vi "xml_set_target.vi"(2 "error in (no error)":errorcluster, 3 "XML Path":path=path "D:/Test Management/Farmer/XML/targets.xml", 4 "Data":T1) -> (0 "error out":errorcluster, 1 "success?":bool)   [LabVIEW 2011]
uses:
  TargetData.ctl
  <vilib>/xml/Load XML File.vi
  <vilib>/xml/Close Reference(Node).vi
  <vilib>/xml/NI_XML.lvlib
  Program Files/National Instruments/LabVIEW 2011/resource/objmgr/DOMUserDefRef.rc
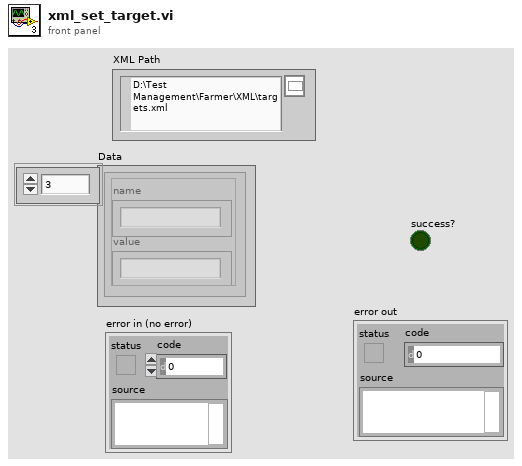
[diagram p1: front panel]
types:
  T1 = typedef "TargetData.ctl" = cluster{"name":string, "value":string}[]
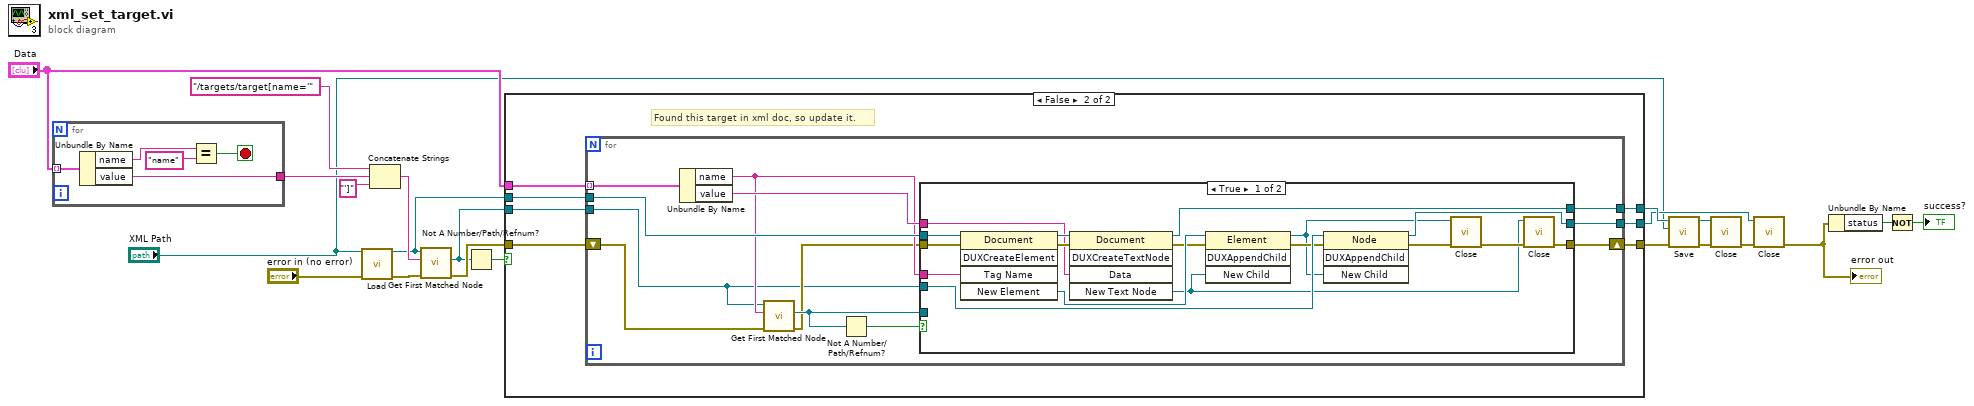
[diagram p0: block diagram]
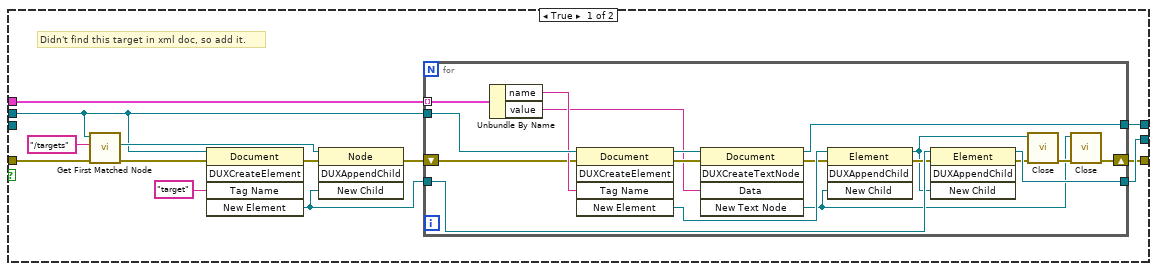
[diagram p2: hidden frame]
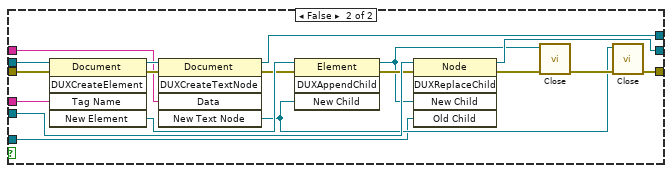
[diagram p3: hidden frame]
diagram:
  n1 = for {
    tunnel: "Data" -> [w26] mode=indexing
    tunnel: [w22] -> w14
    stop <- w23 stop-if-true
    n2 = Unbundle By Name(w26) -> ("name"=w25:string, "value"=w22:string)
    n3 = Equal?(x=w25, y="name") -> (x = y?=w23:bool)
  }
  n4 = call-poly <vilib>:"Load.vi"("path to XML document"="XML Path", "error in (no error)"="error in (no error)") -> ("DOM document out"=w15:refnum<k20>, "error out"=w18:errorcluster)  [unwired: 11 in, 1 out]
  n5 = Concatenate Strings("/targets/target[name='", w14, "']") -> (w19:string)
  n6 = call <vilib>:"Get First Matched Node.vi"("error in (no error)"=w18, "XPath expression"=w19, "node in"=w15) -> ("error out"=w17:errorcluster, "node result"=w6:refnum<k20>)  [unwired: 6 in, 1 out]
  n7 = Not A Number/Path/Refnum?(number/path/refnum=w6) -> (NaN/Path/Refnum?=w16:bool)
  n8 = case shown="False" w16 {
    tunnel: w17 -> [w36 w60]
    tunnel: w15 -> [w29 w63]
    tunnel: "Data" -> [w38 w64]
    tunnel: [w27 w61] -> w12
    tunnel: [w28 w62] -> w11
    tunnel: [w30 w58] -> w10
    tunnel: w6 -> [_ w59]
    frame True {
      # "Didn't find this target in xml doc, so add it."
      n9 = call <vilib>:"Get First Matched Node.vi"("error in (no error)"=w36, "XPath expression"="/targets", "node in"=w29) -> ("error out"=w35:errorcluster, "node result"=w31:refnum<k20>)  [unwired: 6 in, 1 out]
      n10 = invoke class="Document" method="DUXCreateElement"(reference=w29, error in=w35, "Tag Name"="target" ("Data")) -> (error out=w34:errorcluster, "New Element"=w32:refnum<k20>)  [unwired: 2 in, 3 out]
      n11 = invoke class="Node" method="DUXAppendChild"(reference=w31, error in=w34, "New Child"=w32) -> (error out=w33:errorcluster)  [unwired: 1 in, 3 out]
      n12 = for {
        tunnel: w38 -> [w56] mode=indexing
        tunnel: w29 -> [w57]
        shift-right: [w42] -> w27
        shift-left: w33 -> [w53]
        tunnel: [w45] -> w28
        tunnel: w32 -> [w54]
        tunnel: [w52] -> w30
        n13 = Unbundle By Name(w56) -> ("name"=w55:string, "value"=w49:string)
        n14 = invoke class="Document" method="DUXCreateElement"(reference=w57, error in=w53, "Tag Name"=w55) -> (reference out=w51:refnum<k20>, error out=w50:errorcluster, "New Element"=w47:refnum<k20>)  [unwired: 2 in, 2 out]
        n15 = invoke class="Document" method="DUXCreateTextNode"(reference=w51, error in=w50, "Data"=w49) -> (reference out=w45:refnum<k20>, error out=w46:errorcluster, "New Text Node"=w40:refnum<k20>)  [unwired: 2 in, 2 out]
        n16 = invoke class="Element" method="DUXAppendChild"(reference=w47, error in=w46, "New Child"=w40) -> (reference out=w41:refnum<k20>, error out=w48:errorcluster)  [unwired: 1 in, 2 out]
        n17 = invoke class="Element" method="DUXAppendChild"(reference=w54, error in=w48, "New Child"=w41) -> (reference out=w52:refnum<k20>, error out=w44:errorcluster)  [unwired: 1 in, 2 out]
        n18 = call-poly <vilib>:"Close.vi"("error in (no error)"=w44, "node"=w41) -> ("error out"=w43:errorcluster)  [unwired: 7 in]
        n19 = call-poly <vilib>:"Close.vi"("error in (no error)"=w43, "node"=w40) -> ("error out"=w42:errorcluster)  [unwired: 7 in]
      }
    }
    frame False {
      # "Found this target in xml doc, so update it."
      n20 = for {
        tunnel: w64 -> [w75] mode=indexing
        tunnel: w63 -> [w76]
        shift-right: [w73] -> w61
        shift-left: w60 -> [w72]
        tunnel: [w74] -> w62
        tunnel: w59 -> [w66]
        tunnel: [w65] -> w58
        n21 = Unbundle By Name(w75) -> ("name"=w69:string, "value"=w71:string)
        n22 = call <vilib>:"Get First Matched Node.vi"("error in (no error)"=w72, "XPath expression"=w69, "node in"=w66) -> ("error out"=w67:errorcluster, "node result"=w68:refnum<k20>)  [unwired: 6 in, 1 out]
        n23 = Not A Number/Path/Refnum?(number/path/refnum=w68) -> (NaN/Path/Refnum?=w70:bool)
        n24 = case shown="True" w70 {
          tunnel: w76 -> [w93 w111]
          tunnel: w66 -> [w92 w110]
          tunnel: [w91 w109] -> w65
          tunnel: [w85 w103] -> w74
          tunnel: [w82 w100] -> w73
          tunnel: w71 -> [w79 w97]
          tunnel: w69 -> [w78 w96]
          tunnel: w68 -> [_ w95]
          tunnel: w67 -> [w77 w94]
          frame True {
            n25 = invoke class="Document" method="DUXCreateElement"(reference=w93, error in=w77, "Tag Name"=w78) -> (reference out=w90:refnum<k20>, error out=w89:errorcluster, "New Element"=w87:refnum<k20>)  [unwired: 2 in, 2 out]
            n26 = invoke class="Document" method="DUXCreateTextNode"(reference=w90, error in=w89, "Data"=w79) -> (reference out=w85:refnum<k20>, error out=w86:errorcluster, "New Text Node"=w80:refnum<k20>)  [unwired: 2 in, 2 out]
            n27 = invoke class="Element" method="DUXAppendChild"(reference=w87, error in=w86, "New Child"=w80) -> (reference out=w81:refnum<k20>, error out=w88:errorcluster)  [unwired: 1 in, 2 out]
            n28 = invoke class="Node" method="DUXAppendChild"(reference=w92, error in=w88, "New Child"=w81) -> (reference out=w91:refnum<k20>, error out=w84:errorcluster)  [unwired: 1 in, 2 out]
            n29 = call-poly <vilib>:"Close.vi"("error in (no error)"=w84, "node"=w81) -> ("error out"=w83:errorcluster)  [unwired: 7 in]
            n30 = call-poly <vilib>:"Close.vi"("error in (no error)"=w83, "node"=w80) -> ("error out"=w82:errorcluster)  [unwired: 7 in]
          }
          frame False {
            n31 = invoke class="Document" method="DUXCreateElement"(reference=w111, error in=w94, "Tag Name"=w96) -> (reference out=w108:refnum<k20>, error out=w107:errorcluster, "New Element"=w105:refnum<k20>)  [unwired: 2 in, 2 out]
            n32 = invoke class="Document" method="DUXCreateTextNode"(reference=w108, error in=w107, "Data"=w97) -> (reference out=w103:refnum<k20>, error out=w104:errorcluster, "New Text Node"=w98:refnum<k20>)  [unwired: 2 in, 2 out]
            n33 = invoke class="Element" method="DUXAppendChild"(reference=w105, error in=w104, "New Child"=w98) -> (reference out=w99:refnum<k20>, error out=w106:errorcluster)  [unwired: 1 in, 2 out]
            n34 = invoke class="Node" method="DUXReplaceChild"(reference=w110, error in=w106, "New Child"=w99, "Old Child"=w95) -> (reference out=w109:refnum<k20>, error out=w102:errorcluster)  [unwired: 1 in, 3 out]
            n35 = call-poly <vilib>:"Close.vi"("error in (no error)"=w102, "node"=w99) -> ("error out"=w101:errorcluster)  [unwired: 7 in]
            n36 = call-poly <vilib>:"Close.vi"("error in (no error)"=w101, "node"=w98) -> ("error out"=w100:errorcluster)  [unwired: 7 in]
          }
        }
      }
    }
  }
  n37 = call <vilib>:"Save.vi"("error in (no error)"=w12, "XML file path"="XML Path", "DOM document in"=w11) -> ("error out"=w8:errorcluster, "DOM document out"=w7:refnum<k20>)  [unwired: 6 in, 1 out]
  n38 = call-poly <vilib>:"Close.vi"("error in (no error)"=w8, "node"=w7) -> ("error out"=w9:errorcluster)  [unwired: 7 in]
  n39 = call-poly <vilib>:"Close.vi"("error in (no error)"=w9, "node"=w10) -> ("error out"=w4:errorcluster)  [unwired: 7 in]
  "error out" <- w4
  n40 = Unbundle By Name(w4) -> ("status"=w3:bool)
  n41 = Not(x=w3) -> (.not. x?=→"success?":bool)
